vi "recivir_datos.vi"() -> ()   [LabVIEW 2025]
uses:
  <vilib>/httpClient/PUTBuffer.vi
  <vilib>/httpClient/LabVIEWHTTPClient.lvlib
panel:
  in  "Tab Control":T1(tab)
  in  "dt":dbl
  in  "ki":dbl
  in  "kd":dbl
  in  "enviar datos 2":bool
  out "error PUT 2":errorcluster
  out "headers PUT 2":string
  out "body PUT 2":string
  in  "Set-Point":dbl
  in  "Sensor":dbl
  in  "RPM 3":dbl
  in  "KI 3":dbl
  in  "KP 3":dbl
  in  "enviar datos 3":bool
  out "error PUT 3":errorcluster
  out "headers PUT 3":string
  out "body PUT 3":string
  in  "kd":dbl
  in  "k":dbl
  in  "ki":dbl
  out "error PUT 4":errorcluster
  out "body PUT 4":string
  out "headers PUT 4":string
  in  "enviar datos 4":bool
  in  "SetPoint":dbl
  in  "enviar datos 5":bool
  in  "RPM":dbl
  in  "KI":dbl
  in  "KP":dbl
  out "error PUT 5":errorcluster
  out "body PUT 5":string
  out "headers PUT 5":string
  in  "sp":dbl
  in  "ki":dbl
  in  "kd":dbl
  out "error PUT 6":errorcluster
  out "body PUT 6":string
  out "headers PUT 6":string
  in  "enviar datos 6":bool
  in  "kp":dbl
  in  "enviar datos 7":bool
  in  "RPM 7":dbl
  in  "KI 7":dbl
  in  "KP 7":dbl
  out "error PUT 7":errorcluster
  out "body PUT 7":string
  out "headers PUT 7":string
  in  "RPM":dbl
  in  "KP":dbl
  in  "KI":dbl
  in  "enviar datos":bool
  out "body PUT":string
  out "headers PUT":string
  out "error PUT":errorcluster
  in  "stop":bool
  # "Unidad Profesional Interdisciplinaria de Ingeniería, Campus Zacatecas"
  # "Titular de la materia: Ramón Jaramillo Martínez"
  # "Elaborado por:\nMaría Jimena Júnez Huerta\nJet Ming Adrián Huang Sánchez\nJesús Said Zesati Márquez"
  # "24/05/2025"
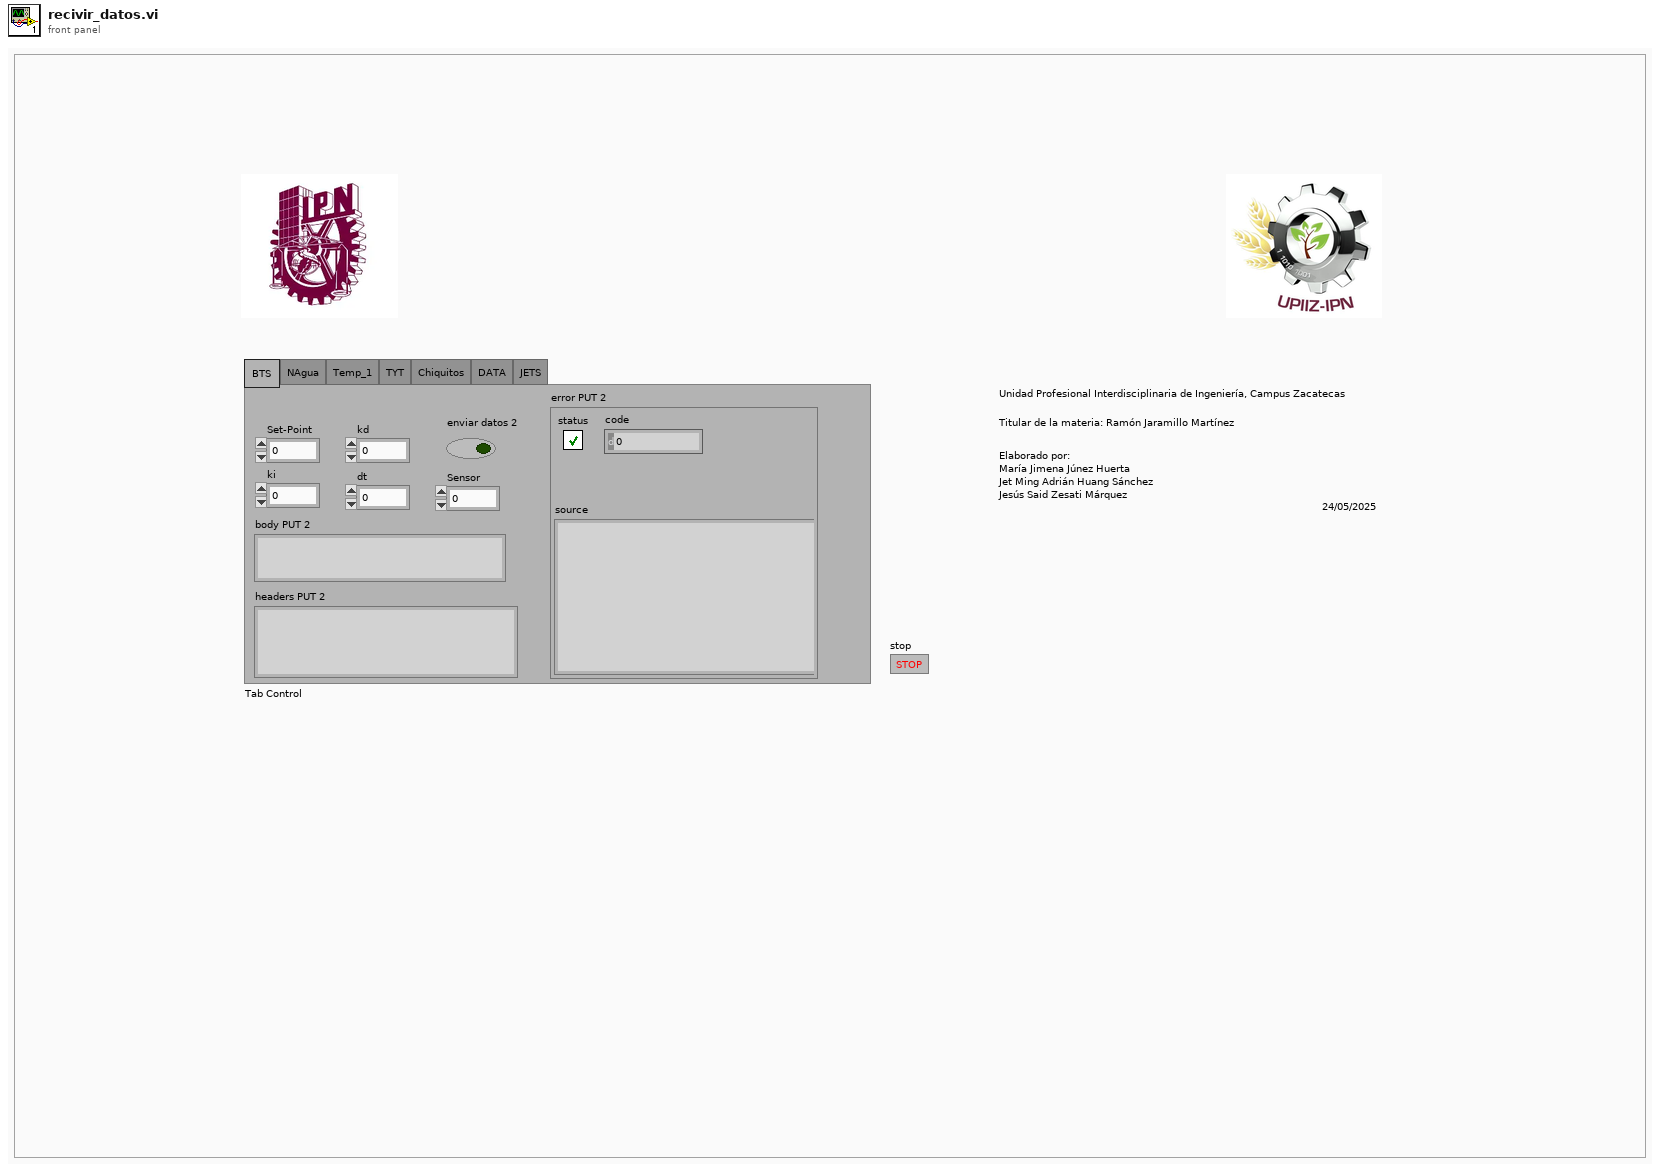
[diagram p1: front panel]
types:
  T1 = enum32{"BTS ", "NAgua", "Temp_1", "TYT", "Chiquitos", "DATA", "JETS"}
  T2 = cluster{"kd":dbl, "ki":dbl, "dt":dbl, "Set-Point":dbl, "Sensor":dbl}
  T3 = cluster{"ki":dbl, "k":dbl, "kd":dbl, "SetPoint":dbl}
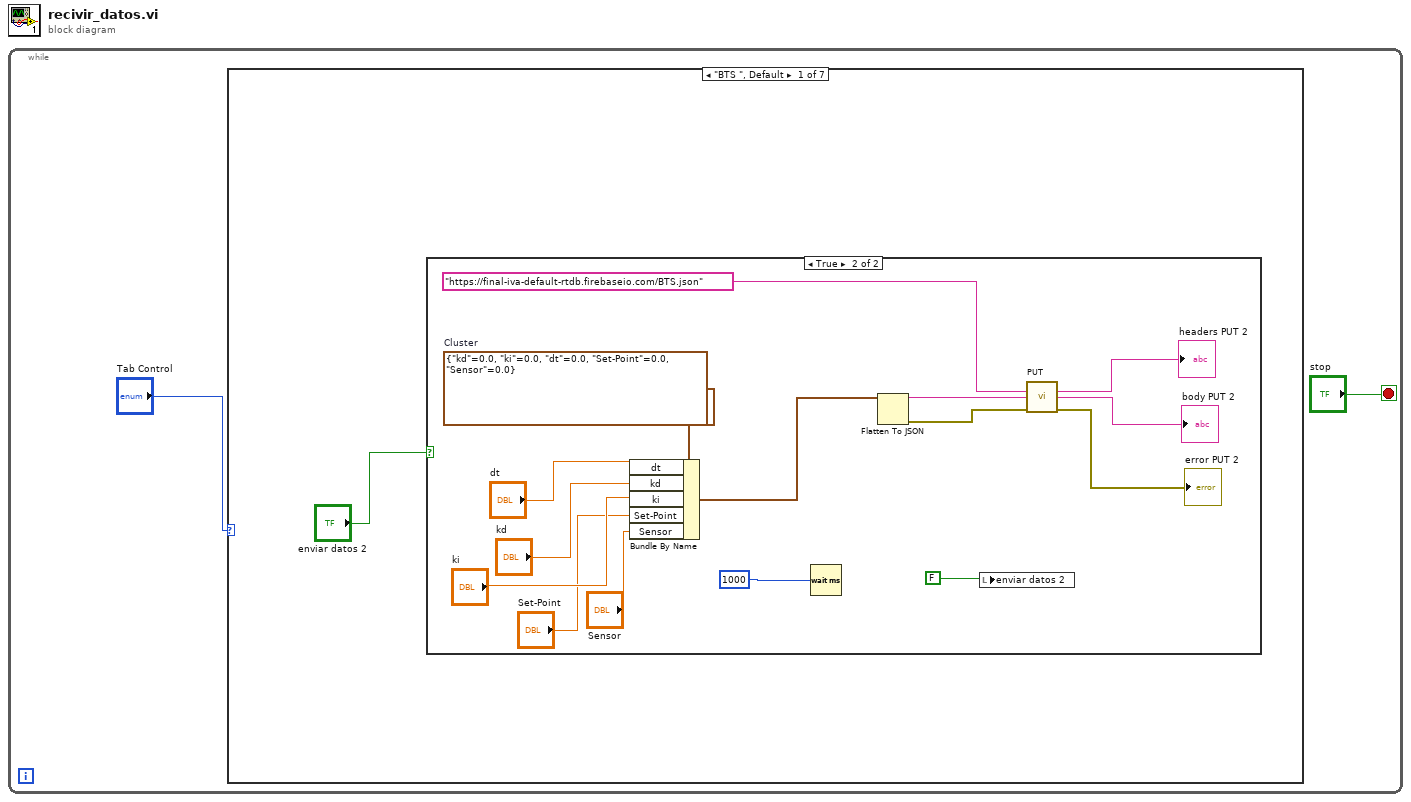
[diagram p0: block diagram]
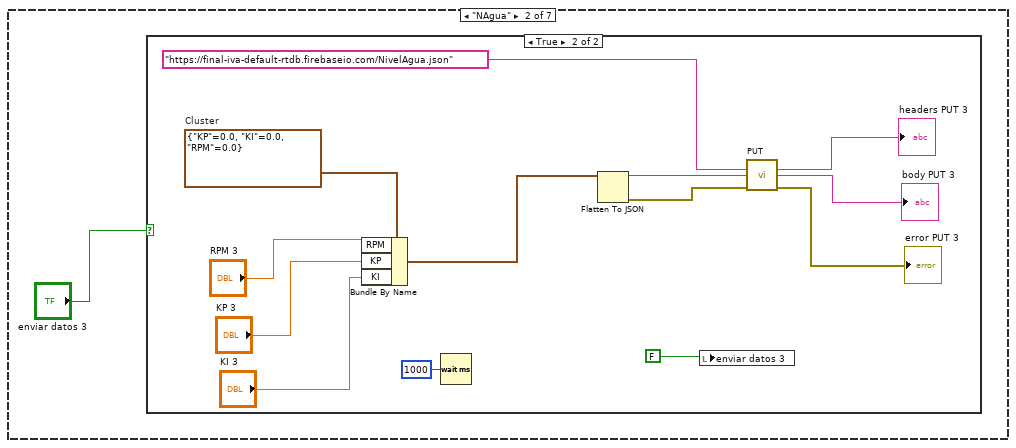
[diagram p3: hidden frame]
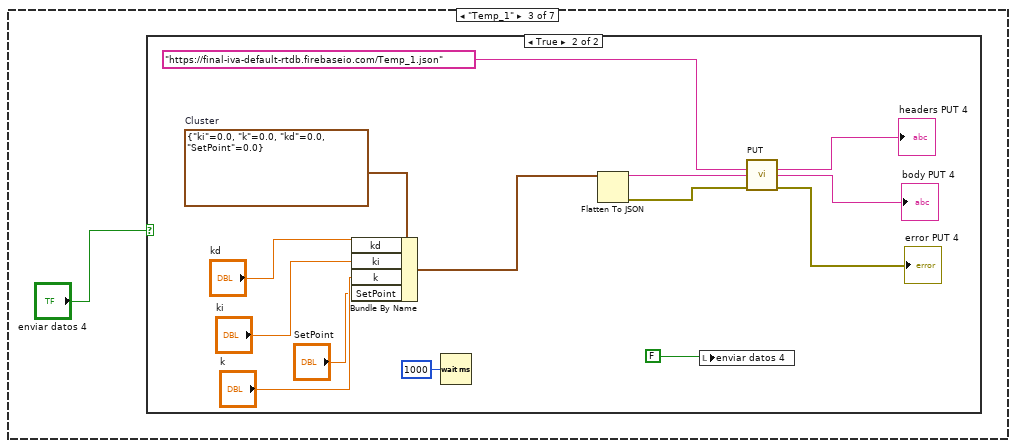
[diagram p5: hidden frame]
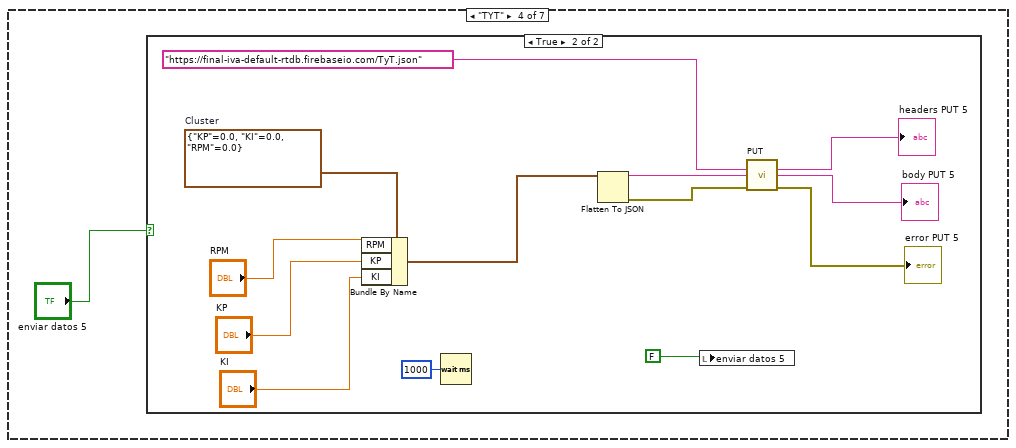
[diagram p7: hidden frame]
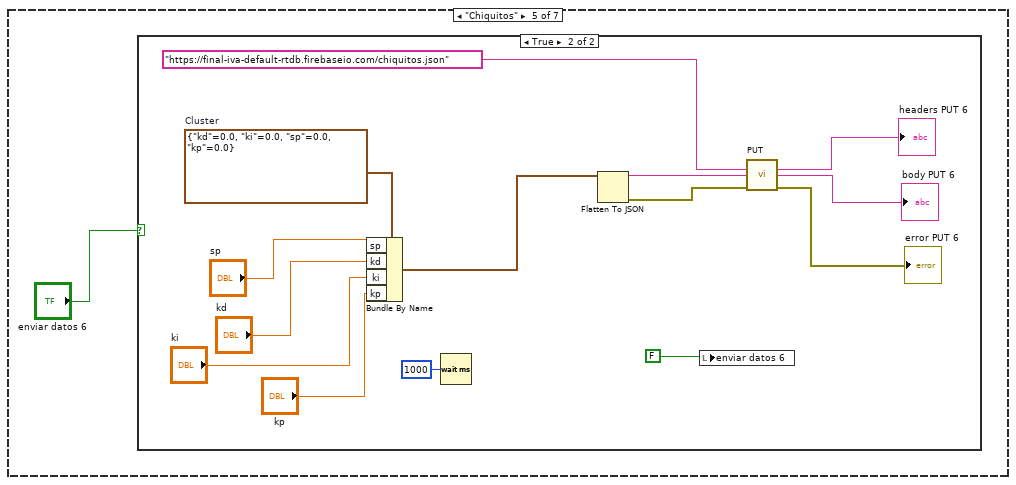
[diagram p9: hidden frame]
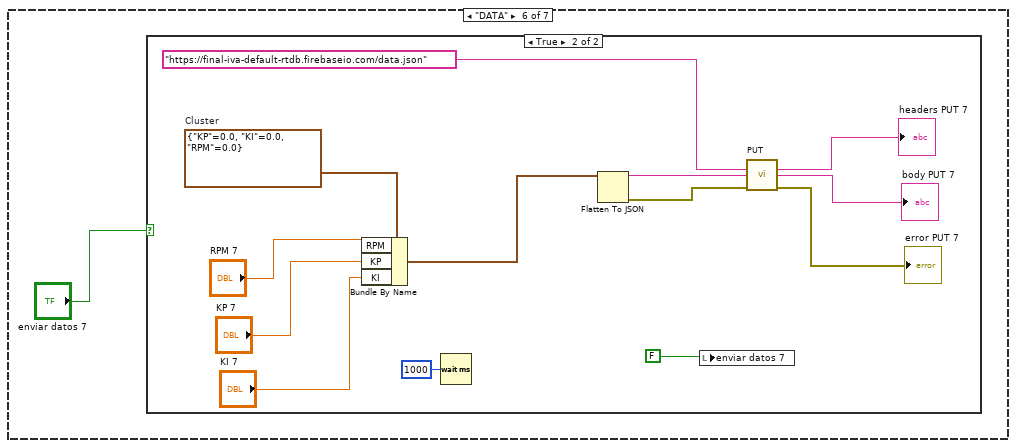
[diagram p11: hidden frame]
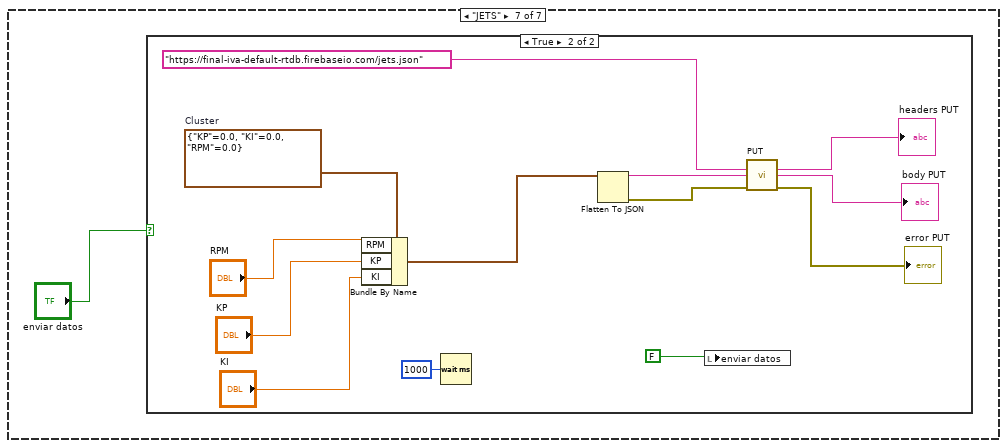
[diagram p13: hidden frame]
diagram:
  n1 = while {
    stop <- "stop" stop-if-true
    n2 = case shown="\"BTS \", Default" "Tab Control" {
      frame "BTS ", Default {
        n3 = case shown="True" "enviar datos 2" {
          frame False {
          }
          frame True {
            w6 = T2 {"kd"=0.0, "ki"=0.0, "dt"=0.0, "Set-Point"=0.0, "Sensor"=0.0}  # Cluster
            n4 = Bundle By Name "Bundle By Name"(cluster=w6, "dt"="dt", "kd"="kd", "ki"="ki", "Set-Point"="Set-Point", "Sensor"="Sensor") -> (w18:T2)
            n5 = Wait (ms)(milliseconds to wait=u32 1000) -> ()  [unwired: 1 out]
            n6 = Flatten To JSON(anything=w18) -> (JSON string=w15:string, 11:w11:errorcluster)  [unwired: 2 in]
            n7 = local write "enviar datos 2"(FALSE) -> ()
            n8 = call-poly <vilib>:"PUT.vi"("url"="https://final-iva-default-rtdb.firebaseio.com/BTS.json", "buffer"=w15, "error in (no error)"=w11) -> ("headers"=→"headers PUT 2":string, "body"=→"body PUT 2":string, "error out"=→"error PUT 2":errorcluster)  [unwired: 9 in, 1 out]
          }
        }
      }
      frame "NAgua" {
        n9 = case shown="True" "enviar datos 3" {
          frame False {
          }
          frame True {
            w26 = cluster{"KP":dbl, "KI":dbl, "RPM":dbl} {"KP"=0.0, "KI"=0.0, "RPM"=0.0}  # Cluster
            n10 = Bundle By Name "Bundle By Name"(cluster=w26, "RPM"="RPM 3", "KP"="KP 3", "KI"="KI 3") -> (w32:cluster{"KP":dbl, "KI":dbl, "RPM":dbl})
            n11 = Wait (ms)(milliseconds to wait=u32 1000) -> ()  [unwired: 1 out]
            n12 = Flatten To JSON(anything=w32) -> (JSON string=w29:string, 11:w24:errorcluster)  [unwired: 2 in]
            n13 = local write "enviar datos 3"(FALSE) -> ()
            n14 = call-poly <vilib>:"PUT.vi"("url"="https://final-iva-default-rtdb.firebaseio.com/NivelAgua.json", "buffer"=w29, "error in (no error)"=w24) -> ("headers"=→"headers PUT 3":string, "body"=→"body PUT 3":string, "error out"=→"error PUT 3":errorcluster)  [unwired: 9 in, 1 out]
          }
        }
      }
      frame "Temp_1" {
        n15 = case shown="True" "enviar datos 4" {
          frame False {
          }
          frame True {
            w41 = T3 {"ki"=0.0, "k"=0.0, "kd"=0.0, "SetPoint"=0.0}  # Cluster
            n16 = Bundle By Name "Bundle By Name"(cluster=w41, "kd"="kd", "ki"="ki", "k"="k", "SetPoint"="SetPoint") -> (w47:T3)
            n17 = Wait (ms)(milliseconds to wait=u32 1000) -> ()  [unwired: 1 out]
            n18 = Flatten To JSON(anything=w47) -> (JSON string=w44:string, 11:w39:errorcluster)  [unwired: 2 in]
            n19 = local write "enviar datos 4"(FALSE) -> ()
            n20 = call-poly <vilib>:"PUT.vi"("url"="https://final-iva-default-rtdb.firebaseio.com/Temp_1.json", "buffer"=w44, "error in (no error)"=w39) -> ("headers"=→"headers PUT 4":string, "body"=→"body PUT 4":string, "error out"=→"error PUT 4":errorcluster)  [unwired: 9 in, 1 out]
          }
        }
      }
      frame "TYT" {
        n21 = case shown="True" "enviar datos 5" {
          frame False {
          }
          frame True {
            w55 = cluster{"KP":dbl, "KI":dbl, "RPM":dbl} {"KP"=0.0, "KI"=0.0, "RPM"=0.0}  # Cluster
            n22 = Bundle By Name "Bundle By Name"(cluster=w55, "RPM"="RPM", "KP"="KP", "KI"="KI") -> (w61:cluster{"KP":dbl, "KI":dbl, "RPM":dbl})
            n23 = Wait (ms)(milliseconds to wait=u32 1000) -> ()  [unwired: 1 out]
            n24 = Flatten To JSON(anything=w61) -> (JSON string=w58:string, 11:w53:errorcluster)  [unwired: 2 in]
            n25 = local write "enviar datos 5"(FALSE) -> ()
            n26 = call-poly <vilib>:"PUT.vi"("url"="https://final-iva-default-rtdb.firebaseio.com/TyT.json", "buffer"=w58, "error in (no error)"=w53) -> ("headers"=→"headers PUT 5":string, "body"=→"body PUT 5":string, "error out"=→"error PUT 5":errorcluster)  [unwired: 9 in, 1 out]
          }
        }
      }
      frame "Chiquitos" {
        n27 = case shown="True" "enviar datos 6" {
          frame False {
          }
          frame True {
            w70 = cluster{"kd":dbl, "ki":dbl, "sp":dbl, "kp":dbl} {"kd"=0.0, "ki"=0.0, "sp"=0.0, "kp"=0.0}  # Cluster
            n28 = Bundle By Name "Bundle By Name"(cluster=w70, "sp"="sp", "kd"="kd", "ki"="ki", "kp"="kp") -> (w76:cluster{"kd":dbl, "ki":dbl, "sp":dbl, "kp":dbl})
            n29 = Wait (ms)(milliseconds to wait=u32 1000) -> ()  [unwired: 1 out]
            n30 = Flatten To JSON(anything=w76) -> (JSON string=w73:string, 11:w68:errorcluster)  [unwired: 2 in]
            n31 = local write "enviar datos 6"(FALSE) -> ()
            n32 = call-poly <vilib>:"PUT.vi"("url"="https://final-iva-default-rtdb.firebaseio.com/chiquitos.json", "buffer"=w73, "error in (no error)"=w68) -> ("headers"=→"headers PUT 6":string, "body"=→"body PUT 6":string, "error out"=→"error PUT 6":errorcluster)  [unwired: 9 in, 1 out]
          }
        }
      }
      frame "DATA" {
        n33 = case shown="True" "enviar datos 7" {
          frame False {
          }
          frame True {
            w84 = cluster{"KP":dbl, "KI":dbl, "RPM":dbl} {"KP"=0.0, "KI"=0.0, "RPM"=0.0}  # Cluster
            n34 = Bundle By Name "Bundle By Name"(cluster=w84, "RPM"="RPM 7", "KP"="KP 7", "KI"="KI 7") -> (w90:cluster{"KP":dbl, "KI":dbl, "RPM":dbl})
            n35 = Wait (ms)(milliseconds to wait=u32 1000) -> ()  [unwired: 1 out]
            n36 = Flatten To JSON(anything=w90) -> (JSON string=w87:string, 11:w82:errorcluster)  [unwired: 2 in]
            n37 = local write "enviar datos 7"(FALSE) -> ()
            n38 = call-poly <vilib>:"PUT.vi"("url"="https://final-iva-default-rtdb.firebaseio.com/data.json", "buffer"=w87, "error in (no error)"=w82) -> ("headers"=→"headers PUT 7":string, "body"=→"body PUT 7":string, "error out"=→"error PUT 7":errorcluster)  [unwired: 9 in, 1 out]
          }
        }
      }
      frame "JETS" {
        n39 = case shown="True" "enviar datos" {
          frame False {
          }
          frame True {
            w98 = cluster{"KP":dbl, "KI":dbl, "RPM":dbl} {"KP"=0.0, "KI"=0.0, "RPM"=0.0}  # Cluster
            n40 = Bundle By Name "Bundle By Name"(cluster=w98, "RPM"="RPM", "KP"="KP", "KI"="KI") -> (w104:cluster{"KP":dbl, "KI":dbl, "RPM":dbl})
            n41 = Wait (ms)(milliseconds to wait=u32 1000) -> ()  [unwired: 1 out]
            n42 = Flatten To JSON(anything=w104) -> (JSON string=w101:string, 11:w96:errorcluster)  [unwired: 2 in]
            n43 = local write "enviar datos"(FALSE) -> ()
            n44 = call-poly <vilib>:"PUT.vi"("url"="https://final-iva-default-rtdb.firebaseio.com/jets.json", "buffer"=w101, "error in (no error)"=w96) -> ("headers"=→"headers PUT":string, "body"=→"body PUT":string, "error out"=→"error PUT":errorcluster)  [unwired: 9 in, 1 out]
          }
        }
      }
    }
  }
